vi "NewGame.vi"(8 "error in (no error)":errorcluster, 10 "Engine in":refnum<class "Engine.lvclass">, 11 "SnakeDemoType (ChildObject)":refnum<class "SnakeDemo.lvclass">) -> (0 "error out":errorcluster, 2 "Engine out":refnum<class "Engine.lvclass">, 3 "SnakeDemo out":refnum<class "SnakeDemo.lvclass">)   [LabVIEW 2019, in "RT_Game.lvlib" / "SnakeDemo.lvclass"]
uses:
  SnakeDemo.lvclass
  C:/Users/FreshBob/Dropbox/VIs/myRIO_GameConsole/RT/RT_Game/Game/Game.lvclass
  C:/Users/FreshBob/Dropbox/VIs/myRIO_GameConsole/RT/RT_Game/SnakeGame/SnakeGame.lvclass
  Engine/Engine.lvclass
  Game/Game.lvclass/Game.ctl
  SnakeGame/SnakeGame.lvclass/SnakeGame.ctl
  Game/Write Singleplayer.vi
  SnakeGame/Write target_count.vi
  Game/Write HasMenu_.vi
  Game/Write HasHighscore_.vi
  SnakeGame/SnakeGame.lvclass
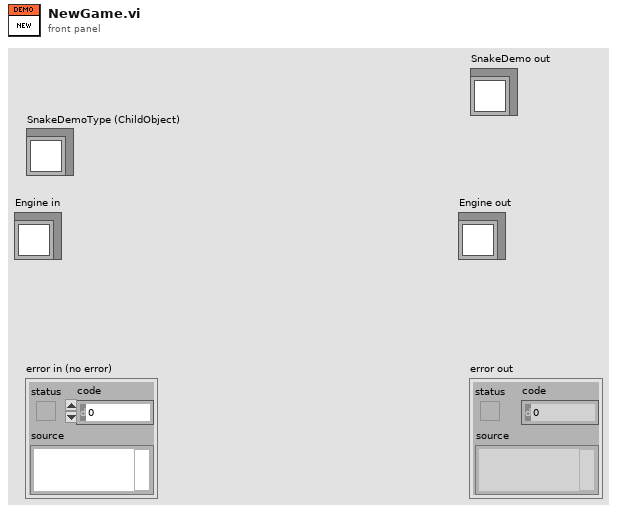
[diagram p1: front panel]
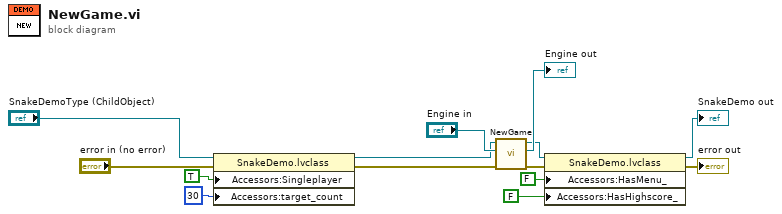
[diagram p0: block diagram]
diagram:
  n1 = property class="SnakeDemo.lvclass"(reference="SnakeDemoType (ChildObject)", error in="error in (no error)", "Accessors:Singleplayer"=TRUE ("Singleplayer"), "Accessors:target_count"=i16 30 ("target_count")) -> (reference out=w9:refnum<class "SnakeDemo.lvclass">, error out=w11:errorcluster)
  n2 = call-parent "NewGame.vi"("error in (no error)"=w11, "Engine in"="Engine in", "SnakeGameType (ChildObject)"=w9) -> ("error out"=w7:errorcluster, "Engine out"=→"Engine out":refnum<class "Engine.lvclass">, "SnakeGame out"=w4:refnum<class "SnakeDemo.lvclass">)  [unwired: 6 in]
  n3 = property class="SnakeDemo.lvclass"(reference=w4, error in=w7, "Accessors:HasMenu_"=FALSE ("HasMenu_"), "Accessors:HasHighscore_"=FALSE ("HasHighscore_")) -> (reference out=→"SnakeDemo out":refnum<class "SnakeDemo.lvclass">, error out=→"error out":errorcluster)
